vi "get name from file extension.vi"(9 "file ext":string, 11 "file name (no ext)":string) -> (1 "extension folder":string, 3 "file name with ext":string)   [LabVIEW 2023, in "File Classes.lvlib"]
uses:
  File Classes.lvlib
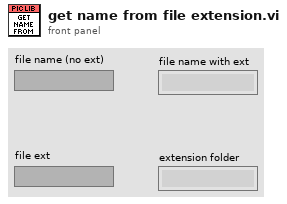
[diagram p1: front panel]
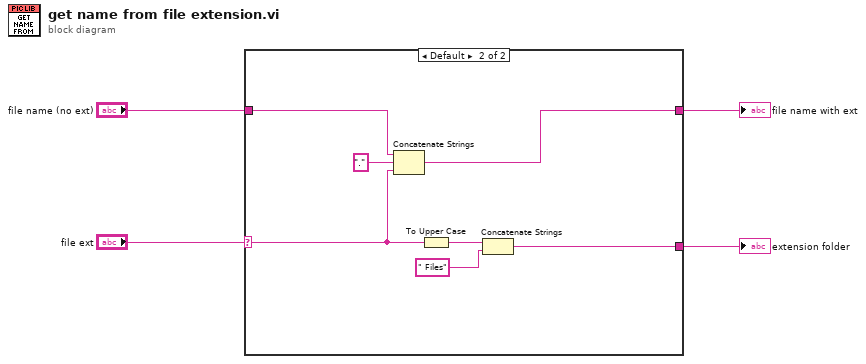
[diagram p0: block diagram]
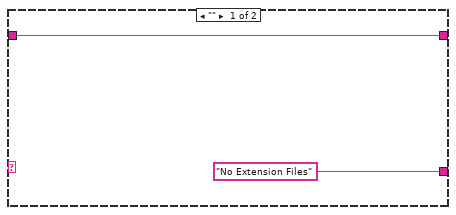
[diagram p2: hidden frame]
diagram:
  n1 = case shown="Default" "file ext" {
    selector: "file ext" -> [_ w11]
    tunnel: "file name (no ext)" -> [w6 w13]
    tunnel: ["No Extension Files" w8] -> w2
    tunnel: [w6 w7] -> w1
    frame "" {
    }
    frame Default {
      n2 = Concatenate Strings(w13, "." ("string"), w11) -> (w7:string)
      n3 = To Upper Case(1:w11) -> (0:w10:string)
      n4 = Concatenate Strings(w10, " Files" ("string")) -> (w8:string)
    }
  }
  "extension folder" <- w2
  "file name with ext" <- w1
